vi "Alarm Clock.vi"() -> ()   [LabVIEW 2020]
uses:
  Selected Clock(Global Variable).vi
panel:
  out "Selected Alarm Clock":timestamp format="%<%X\n%x>T"
  in  "On/Off":bool=TRUE
  out "Date":string
  out "Alarm":bool
  in  "variabe 2":bool
  out "Time":string
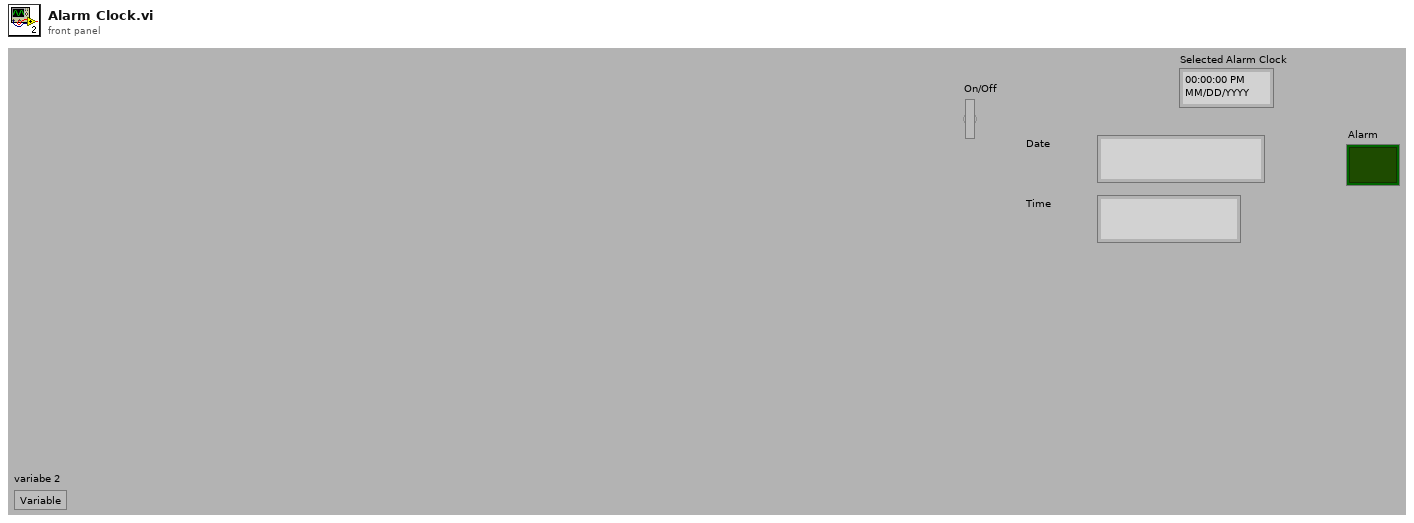
[diagram p1: front panel]
types:
  T1 = enum16{"Left Button", "Center Button", "Right Button", "Window Close"}
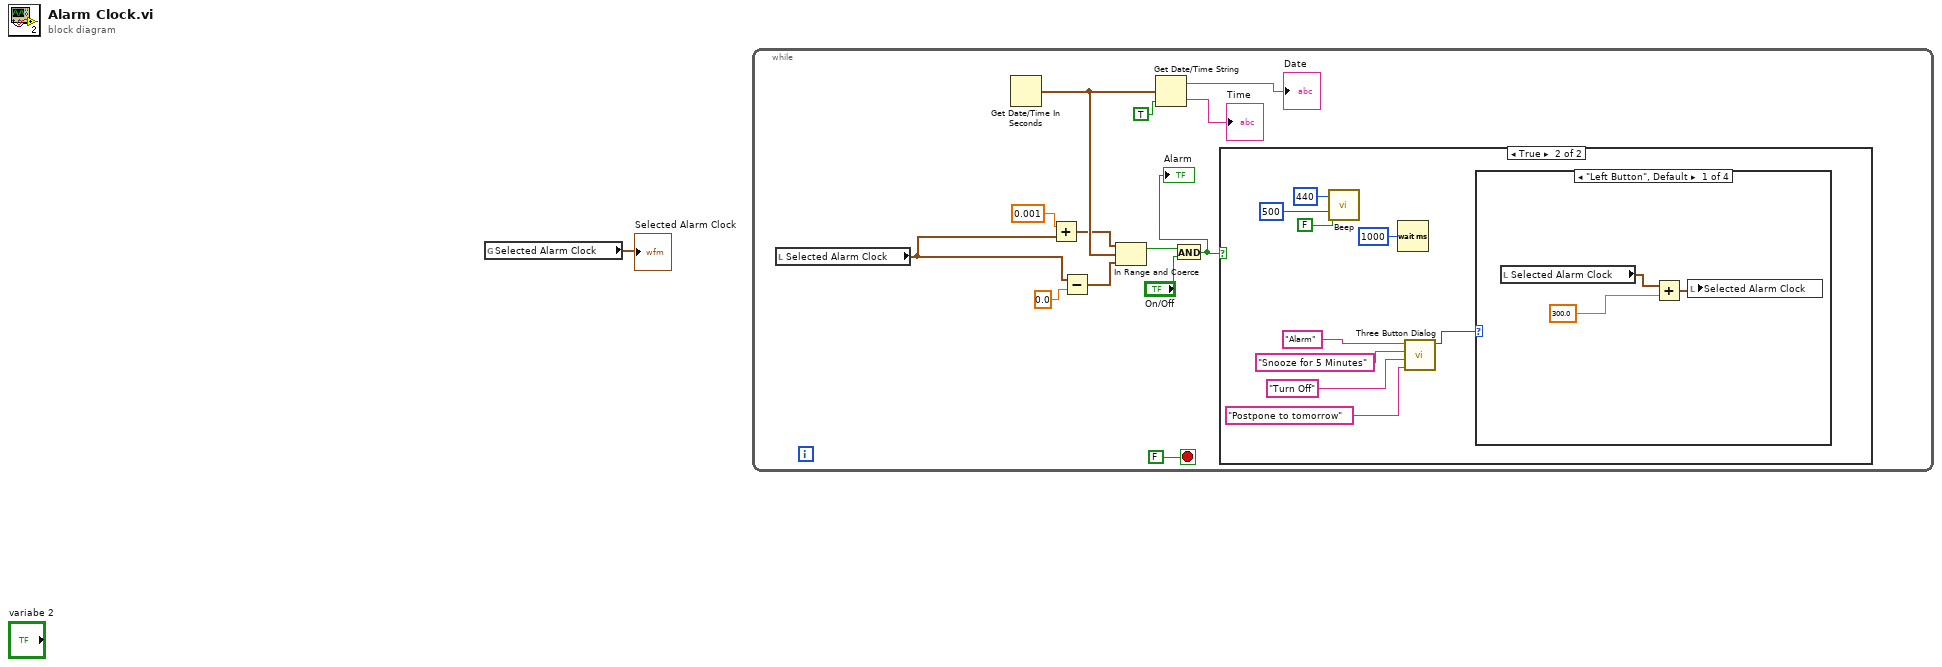
[diagram p0: block diagram]
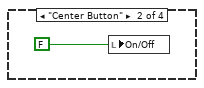
[diagram p3: hidden frame]
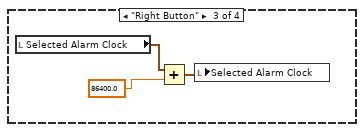
[diagram p4: hidden frame]
diagram:
  n1 = global read "Selected Clock(Global Variable).vi" "Selected Alarm Clock"() -> (→"Selected Alarm Clock":timestamp)
  n2 = while {
    stop <- FALSE stop-if-true
    n3 = local read "Selected Alarm Clock"() -> (w4:timestamp)
    n4 = Get Date/Time In Seconds() -> (seconds since 1Jan1904=w5:timestamp)
    n5 = Add(x=0.001, y=w4) -> (x+y=w3:timestamp)
    n6 = Subtract(x=w4, y=0.0 ("x")) -> (x-y=w2:timestamp)
    n7 = In Range and Coerce(upper limit=w3, x=w5, lower limit=w2) -> (In Range?=w7:bool)  [unwired: 1 out]
    n8 = Get Date/Time String(seconds (now)=w5, want seconds? (F)=TRUE) -> (date string=→"Date":string, time string=→"Time":string)  [unwired: 1 in]
    n9 = And(x=w7, y="On/Off") -> (x .and. y?=w10:bool)
    "Alarm" <- w10
    n10 = case shown="True" w10 {
      frame False {
      }
      frame True {
        n11 = call <vilib>:"Beep.vi"("use system alert? (T)"=FALSE, "duration (msec)"=u32 500, "frequency (Hz)"=u32 440) -> ()  [unwired: 9 in]
        n12 = Wait (ms)(milliseconds to wait=u32 1000) -> ()  [unwired: 1 out]
        n13 = call <vilib>:"Three Button Dialog.vi"("Right Button Text (\"Cancel\")"="Postpone to tomorrow" ("T button name (\"OK\")"), "Center Button Text (\"No\")"="Turn Off" ("T button name (\"OK\")"), "Left Button Text (\"Yes\")"="Snooze for 5 Minutes" ("F button name (\"Cancel\")"), "message"="Alarm") -> ("Which Button?"=w19:T1)  [unwired: 7 in]
        n14 = case shown="\"Left Button\", Default" w19 {
          frame "Left Button", Default {
            n15 = local read "Selected Alarm Clock"() -> (w25:timestamp)
            n16 = Add(x=w25, y=300.0) -> (x+y=w24:timestamp)
            n17 = local write "Selected Alarm Clock"(w24) -> ()
          }
          frame "Center Button" {
            n18 = local write "On/Off"(FALSE ("Boolean")) -> ()
          }
          frame "Right Button" {
            n19 = local read "Selected Alarm Clock"() -> (w29:timestamp)
            n20 = Add(x=w29, y=86400.0) -> (x+y=w28:timestamp)
            n21 = local write "Selected Alarm Clock"(w28) -> ()
          }
          frame "Window Close" {
          }
        }
      }
    }
  }
